vi "报文处理打包.vi"(0 "识别名称":string, 3 "报文":string, 5 "Error In":errorcluster caption="前置通讯错误", 10 "类型":enum16{"被-接收", "被-反馈", "主-发", "主-收"}(ring)) -> (14 "识别名称输出":string, 16 "被收校验信息":cluster{"可用？":bool, "功能码":u8, "无crc报文":u8[]})   [LabVIEW 2019]
panel:
  # "R03\nR06\nR16\nZS\nZR"
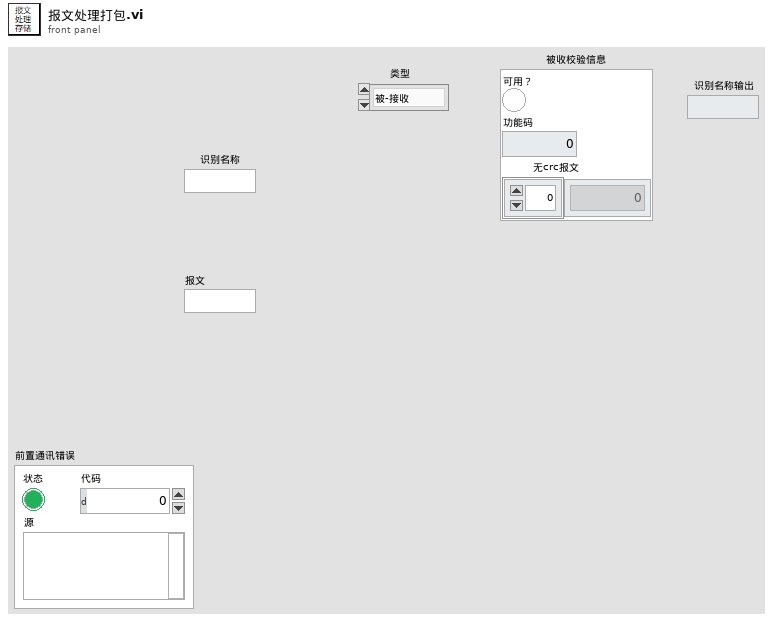
[diagram p1: front panel]
types:
  T1 = enum16{"ini", "增", "删", "查", "改-通讯状态", "改-记录上限", "增-报文", "清空报文记录", "清空全部记录"}
  T2 = cluster{"识别名称":string, "记录":cluster{"通讯状态":bool, "记录上限":dbl, "报文记录":string[]}}
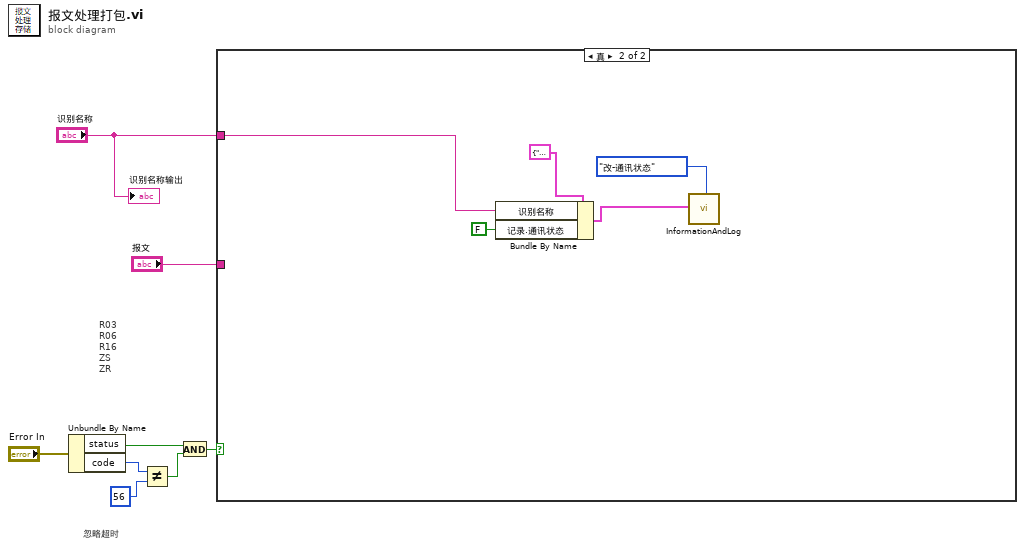
[diagram p0: block diagram]
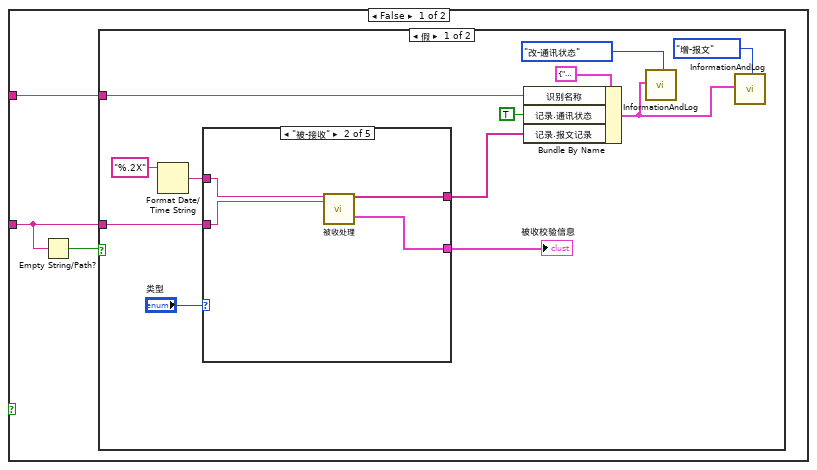
[diagram p2: hidden frame]
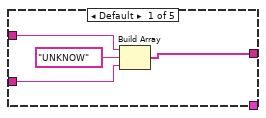
[diagram p3: hidden frame]
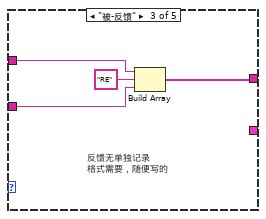
[diagram p4: hidden frame]
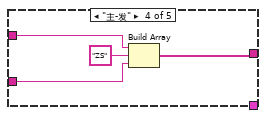
[diagram p5: hidden frame]
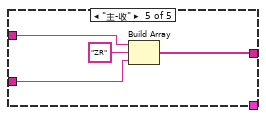
[diagram p6: hidden frame]
diagram:
  # "忽略超时"
  # "R03\nR06\nR16\nZS\nZR"
  n1 = Unbundle By Name("Error In") -> ("status"=w5:bool, "code"=w7:i32)
  n2 = Not Equal?(x=w7, y=56) -> (x != y?=w4:bool)
  n3 = And(x=w5, y=w4) -> (x .and. y?=w3:bool)
  n4 = case shown="真" w3 {
    tunnel: "识别名称" -> [w11 w47]
    tunnel: "报文" -> [w10 _]
    frame False {
      n5 = Empty String/Path?(string/path=w10) -> (empty?=w9:bool)
      n6 = case shown="假" w9 {
        tunnel: w11 -> [w17 _]
        tunnel: w10 -> [w19 _]
        frame False {
          n7 = Format Date/Time String(time format string (%c)="%.2X" ("时间格式字符串(%c)")) -> (date/time string=w20:string)  [unwired: 2 in]
          n8 = case shown="\"被-接收\"" "类型" {
            tunnel: w19 -> [w25 w30 w34 w37 w41]
            tunnel: w20 -> [w26 w31 w35 w38 w42]
            tunnel: [w24 w29 w32 w36 w40] -> w15
            tunnel: [_ w28 _ _ _] -> w12
            frame Default {
              n9 = Build Array(w26, "UNKNOW" ("元素"), w25) -> (w24:string[])
            }
            frame "被-接收" {
              n10 = call "被收处理.vi"("时间"=w31, "报文"=w30) -> ("结果"=w29:string[], "校验信息"=w28:cluster{"可用？":bool, "功能码":u8, "无crc报文":u8[]})  [unwired: 16 in]
            }
            frame "被-反馈" {
              # "反馈无单独记录\n格式需要，随便写的"
              n11 = Build Array(w35, "RE" ("元素"), w34) -> (w32:string[])
            }
            frame "主-发" {
              n12 = Build Array(w38, "ZS" ("元素"), w37) -> (w36:string[])
            }
            frame "主-收" {
              n13 = Build Array(w42, "ZR" ("元素"), w41) -> (w40:string[])
            }
          }
          "被收校验信息" <- w12
          n14 = Bundle By Name(cluster=T2 {"识别名称"="", "记录"={"通讯状态"=FALSE, "记录上限"=0.0, "报文记录"=[]}} ("配置信息"), "识别名称"=w17, "记录.通讯状态"=TRUE, "记录.报文记录"=w15) -> (w14:T2)
          n15 = call "InformationAndLog.vi"("配置信息"=w14, "模拟数据枚举"=T1."改-通讯状态") -> ()  [unwired: 16 in, 2 out]
          n16 = call "InformationAndLog.vi"("配置信息"=w14, "模拟数据枚举"=T1."增-报文") -> ()  [unwired: 16 in, 2 out]
        }
        frame True {
        }
      }
    }
    frame True {
      n17 = Bundle By Name(cluster=T2 {"识别名称"="", "记录"={"通讯状态"=FALSE, "记录上限"=0.0, "报文记录"=[]}} ("配置信息"), "识别名称"=w47, "记录.通讯状态"=FALSE) -> (w45:T2)
      n18 = call "InformationAndLog.vi"("配置信息"=w45, "模拟数据枚举"=T1."改-通讯状态") -> ()  [unwired: 16 in, 2 out]
    }
  }
  "识别名称输出" <- "识别名称"
